vi "Create Employee Table.vi"(8 "错误输入（无错误）":errorcluster, 11 "TableName":string) -> (0 "错误输出":errorcluster, 3 "DataTable Out":refnum<k24>)   [LabVIEW 2012, in "Employee Info.lvlib"]
uses:
  Employee Info.lvlib
  System.Data
  LowLevel/DataGridView.lvlib
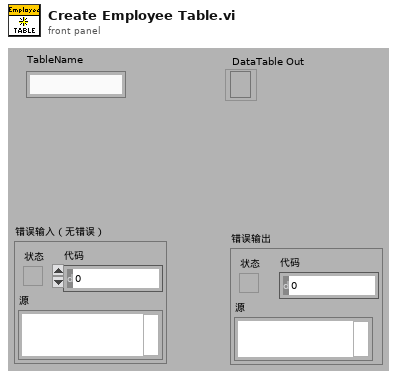
[diagram p1: front panel]
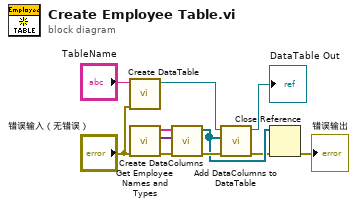
[diagram p0: block diagram]
diagram:
  n1 = call "Create DataTable.vi"("错误输入（无错误）"="错误输入（无错误）", "tableName"="TableName") -> ("DataTable"=w7:refnum<k24>)  [unwired: 8 in, 1 out]
  n2 = call "Get Employee Names and Types.vi"("错误输入（无错误）"="错误输入（无错误）") -> ("错误输出"=w8:errorcluster, "Colomn Types"=w9:variant[], "Column Names"=w10:string[])  [unwired: 8 in]
  n3 = call "Create DataColumns.vi"("错误输入（无错误）"=w8, "DataType"=w9, "ColumnName Array"=w10) -> ("错误输出"=w6:errorcluster, "DataColumns"=w2:refnum<k24>[])  [unwired: 7 in]
  n4 = call "Add DataColumns to DataTable.vi"("错误输入（无错误）"=w6, "DataColumns"=w2, "DataTable"=w7) -> ("错误输出"=w1:errorcluster, "DataTable Out"=→"DataTable Out":refnum<k24>)  [unwired: 7 in]
  n5 = Close Reference(reference=w2, error in (no error)=w1) -> (error out=→"错误输出":errorcluster)
